vi "Command with Return Value.vi"(6 "y":dbl=2.0, 9 "read buffer":string="getAll<6", 10 "Values Read in":dbl[][](array[numeric])=[[200.0, 0.0, 0.0, -99.0, 0.0, 0.0, 0.0], [290.0, 0.0, 0.0, 0.0, 0.0, 0.0, 0.0], [0.0, 0.0, 0.0, 0.0, 0.0, 0.0, 0.0], [0.0, 0.0, 0.0, 0.0, 0.0, 0.0, 0.0], [0.0, 0.0, 0.0, 0.0, 0.0, 0.0, 0.0]], 11 "VISA Refnum in":refnum<visa-resource-name>="ASRL21::INSTR") -> (3 "Values Read out":dbl[][](array[numeric])=[[200.0, 0.0, 0.0, -99.0], [0.0, 290.0, 0.0, 0.0], [0.0, 0.0, 0.0, 0.0], [0.0, 0.0, 0.0, 0.0], [0.0, 0.0, 0.0, 0.0]])   [LabVIEW 2020]
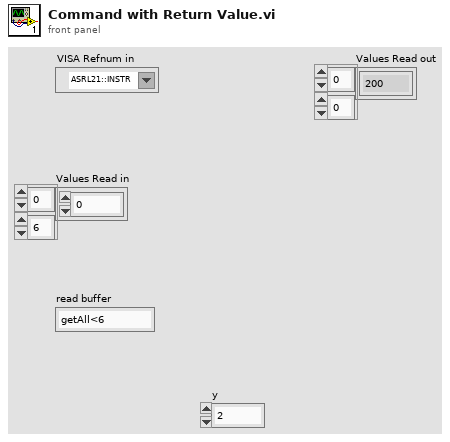
[diagram p1: front panel]
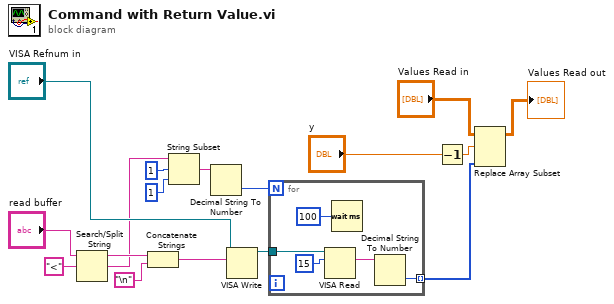
[diagram p0: block diagram]
diagram:
  n1 = Search/Split String(string="read buffer", search string/char (-)="<") -> (substring before match=w11:string, match + rest of string=w7:string)  [unwired: 1 in, 1 out]
  n2 = Concatenate Strings(w11, "\n") -> (w12:string)
  n3 = String Subset(string=w7, offset (0)=1, length (rest)=1 ("length (rest)")) -> (substring=w4:string)
  n4 = Decimal String To Number(string=w4) -> (number=w5:i32)  [unwired: 2 in, 1 out]
  n5 = VISA Write(VISA resource name="VISA Refnum in", write buffer=w12) -> (VISA resource name out=w10:refnum<visa-resource-name>)  [unwired: 1 in, 2 out]
  n6 = for {
    N: w5 -> [_]
    tunnel: w10 -> [w21]
    tunnel: [w18] -> w14 mode=indexing
    n7 = VISA Read(VISA resource name=w21, byte count=u32 15) -> (read buffer=w19:string)  [unwired: 1 in, 3 out]
    n8 = Wait (ms)(milliseconds to wait=u32 100) -> ()  [unwired: 1 out]
    n9 = Decimal String To Number(string=w19) -> (number=w18:i32)  [unwired: 2 in, 1 out]
  }
  n10 = Decrement(x="y") -> (x-1=w16:dbl)
  n11 = Replace Array Subset(array="Values Read in", new element=w14, index (row)=w16) -> (→"Values Read out":dbl[][])  [unwired: 1 in]
